vi "Lab1(Ver2).vi"() -> ()   [LabVIEW 2010]
uses:
  <vilib>/measure/maspectr.llb/FFT Spectrum (Mag-Phase) for 1 Chan.vi
  <vilib>/measure/NI_MABase.lvlib
  <vilib>/measure/NI_MAPro.lvlib
  <vilib>/ptbypt/NI_PtbyPt.lvlib
panel:
  out "power ratio":dbl
  in  "stop":bool
  out "baseband signal (time-domain)":waveform(dbl)(graph)
  out "baseband signal (frequency-domain)":cluster{"f0":dbl, "df":dbl, "magnitude":dbl[]}(graph)
  out "modulated signal (frequency-domain)":cluster{"f0":dbl, "df":dbl, "magnitude":dbl[]}(graph)
  out "modulated signal (time-domain)":waveform(dbl)(graph)
  in  "mod index":dbl(slide)=1.0 scale=0.0..1.0
  in  "modulation frequency":dbl(knob)=10.0 scale=0.0..1000.0
  in  "carrier frequency":dbl(knob)=10.0 scale=0.0..500000.0
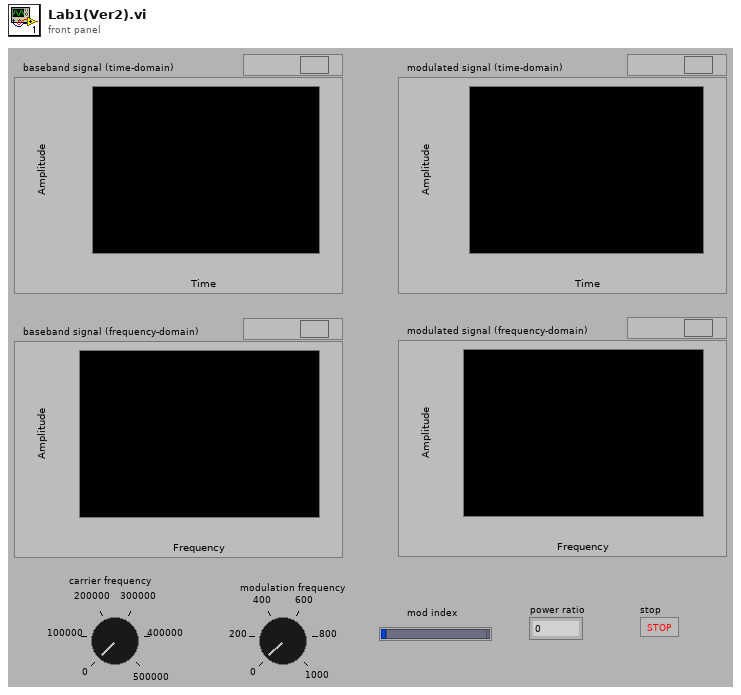
[diagram p1: front panel]
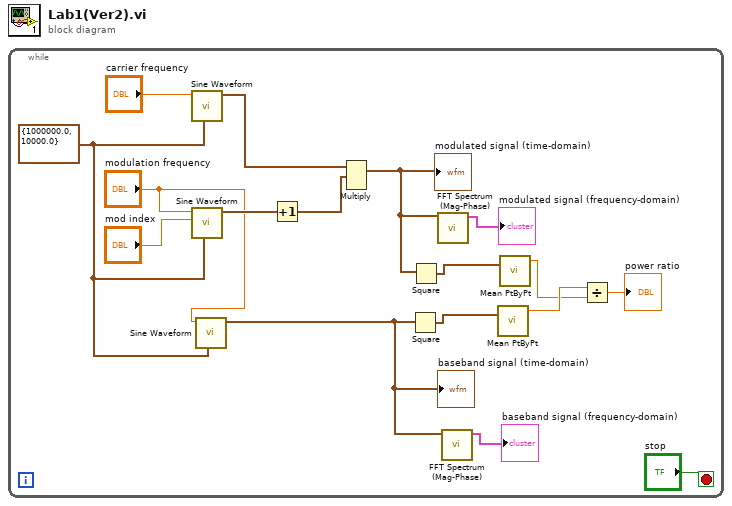
[diagram p0: block diagram]
diagram:
  n1 = while {
    stop <- "stop" stop-if-true
    w1 = cluster{"Fs":dbl, "#s":dbl} {"Fs"=1000000.0, "#s"=10000.0} ("sampling info")
    n2 = call <vilib>:"Sine Waveform.vi"("sampling info"=w1, "frequency"="carrier frequency") -> ("signal out"=w15:waveform(dbl))  [unwired: 8 in, 1 out]
    n3 = call <vilib>:"Sine Waveform.vi"("sampling info"=w1, "amplitude"="mod index", "frequency"="modulation frequency") -> ("signal out"=w6:waveform(dbl))  [unwired: 7 in, 1 out]
    n4 = call <vilib>:"Sine Waveform.vi"("sampling info"=w1, "frequency"="modulation frequency") -> ("signal out"=w3:waveform(dbl))  [unwired: 8 in, 1 out]
    "baseband signal (time-domain)" <- w3
    n5 = Increment(x=w6) -> (x+1=w14:waveform(dbl))
    n6 = Multiply(1:w14, 2:w15) -> (0:w10:waveform(dbl))  [unwired: 1 in, 1 out]
    "modulated signal (time-domain)" <- w10
    n7 = Square(x=w3) -> (x^2=w9:waveform(dbl))
    n8 = Square(x=w10) -> (x^2=w8:waveform(dbl))
    n9 = call-poly <vilib>:"FFT Spectrum (Mag-Phase).vi"("time signal"=w10) -> ("magnitude"=→"modulated signal (frequency-domain)":cluster{"f0":dbl, "df":dbl, "magnitude":dbl[]})  [unwired: 6 in, 4 out]
    n10 = call-poly <vilib>:"FFT Spectrum (Mag-Phase).vi"("time signal"=w3) -> ("magnitude"=→"baseband signal (frequency-domain)":cluster{"f0":dbl, "df":dbl, "magnitude":dbl[]})  [unwired: 6 in, 4 out]
    n11 = call <vilib>:"Mean PtByPt.vi"("x"=w9) -> ("mean"=w5:dbl)  [unwired: 3 in, 1 out]
    n12 = call <vilib>:"Mean PtByPt.vi"("x"=w8) -> ("mean"=w4:dbl)  [unwired: 3 in, 1 out]
    n13 = Divide(x=w5, y=w4) -> (x/y=→"power ratio":dbl)
  }
